vi "Expander Write.vi"(8 "error in (no error)":errorcluster, 9 "Value":u8, 10 "VISA resource name in":refnum<visa-resource-name>, 11 "LCD-I2C in":refnum<class "LCD-I2C.lvclass">) -> (0 "error out":errorcluster, 2 "VISA resource name":refnum<visa-resource-name>, 3 "LCD-I2C out":refnum<class "LCD-I2C.lvclass">)   [LabVIEW 2020, in "CTI-Visa-DeviceLib.lvlib" / "LCD-I2C.lvclass"]
uses:
  LCD-I2C.lvclass
  LCD-I2C.lvclass/LCD-I2C.ctl
  CTI-Visa/CTI-Visa.lvlib
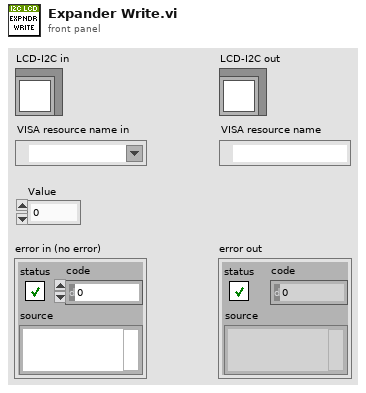
[diagram p1: front panel]
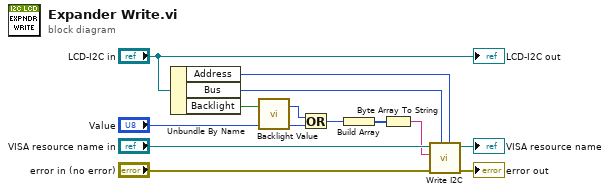
[diagram p0: block diagram]
diagram:
  n1 = Unbundle By Name("LCD-I2C in") -> ("Address"=w7:u8, "Bus"=w6:u8, "Backlight"=w1:bool)
  n2 = call "Backlight Value.vi"("Backlight"=w1) -> ("BacklightVal"=w4:u8)  [unwired: 6 in]
  n3 = Or(x=w4, y="Value") -> (x .or. y?=w2:u8)
  n4 = Build Array(w2) -> (w8:u8[])
  n5 = Byte Array To String(unsigned byte array=w8) -> (string=w5:string)
  n6 = call "Write I2C.vi"("Address"=w7, "Bus"=w6, "error in (no error)"="error in (no error)", "Data"=w5, "VISA resource name in"="VISA resource name in") -> ("error out"=→"error out":errorcluster, "VISA resource name"=→"VISA resource name":refnum<visa-resource-name>)  [unwired: 5 in]
  "LCD-I2C out" <- "LCD-I2C in"
